vi "G# - StaticClassAndClassAttributes.vi"() -> ()   [LabVIEW 2020]
doc: "Static Classes and Class Attributes\nThis example demonstrates how static classes and class attributes works.\n\nBy using the G# Debugger found in Tools->G# Debugger a text log can be followed showing how the objects were created and destroyed."
uses:
  MyOrdinaryClass_class/MyOrdinaryClass.lvclass
  MyStaticClass_class/MyStaticClass.lvclass
  vi.lib/addons/_AddQ/G#Object/G#Object.lvclass
panel:
  in  "error in (no error)":errorcluster
  out "MyClassAttribute after garbage collector":dbl
  out "MyClassAttribute ordinary after garbage collector":string
  out "MyClassAttribute ordinary class unaffected by objects life cycle":string
  out "error out":errorcluster
  out "MyClassAttribute Ordinary Class":string
  out "MyClassAttribute Static Class":dbl
  # "Static Classes and Class Attributes\nThis example demonstrates how static classes and class attributes works.\n\nBy using the G# Debugger found in Tools->G# Debugger a text log can be followed showing how the objects were created and destroyed."
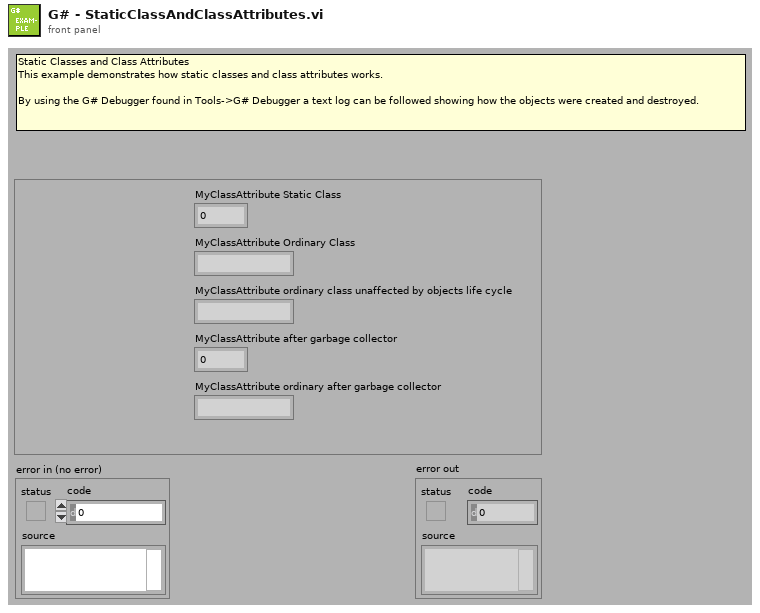
[diagram p1: front panel]
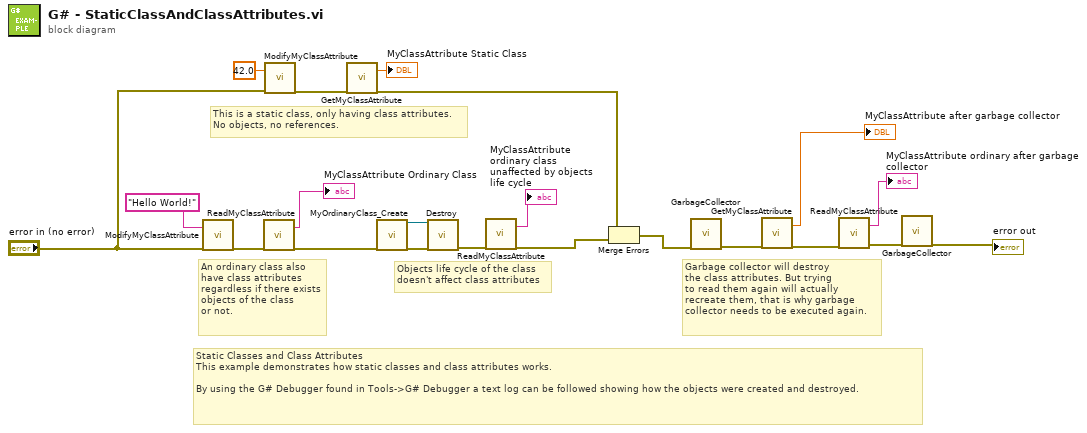
[diagram p0: block diagram]
diagram:
  # "Static Classes and Class Attributes\nThis example demonstrates how static classes and class attributes works.\n\nBy using the G# Debugger found in Tools->G# Debugger a text log can be followed showing how the objects were created and destroyed."
  # "Garbage collector will destroy\nthe class attributes. But trying\nto read them again will actually\nrecreate them, that is why garbage\ncollector needs to be executed again."
  # "Objects life cycle of the class\ndoesn't affect class attributes"
  # "An ordinary class also\nhave class attributes\nregardless if there exists\nobjects of the class\nor not."
  # "This is a static class, only having class attributes.\nNo objects, no references."
  n1 = call "ModifyMyClassAttribute.vi"("string"="Hello World!", "error in (no error)"="error in (no error)") -> ("error out"=w16:errorcluster)  [unwired: 17 in]
  n2 = call "ReadMyClassAttribute.vi"("error in (no error)"=w16) -> ("MyClassAttribute"=→"MyClassAttribute Ordinary Class":string, "error out"=w15:errorcluster)  [unwired: 17 in]
  n3 = call "ModifyMyClassAttribute.vi"("increment"=42.0, "error in (no error)"="error in (no error)") -> ("error out"=w19:errorcluster)  [unwired: 17 in]
  n4 = call "GetMyClassAttribute.vi"("error in (no error)"=w19) -> ("MyClassAttribute"=→"MyClassAttribute Static Class":dbl, "error out"=w17:errorcluster)  [unwired: 17 in]
  n5 = call "MyOrdinaryClass_Create.vi"("error in (no error)"=w15) -> ("reference out"=w13:refnum<class "MyOrdinaryClass.lvclass">, "error out"=w14:errorcluster)  [unwired: 17 in]
  n6 = call-dynamic "Destroy.vi"("reference in"=w13, "error in (no error)"=w14) -> ("error out"=w9:errorcluster)  [unwired: 16 in, 1 out]
  n7 = call "ReadMyClassAttribute.vi"("error in (no error)"=w9) -> ("MyClassAttribute"=→"MyClassAttribute ordinary class unaffected by objects life cycle":string, "error out"=w8:errorcluster)  [unwired: 17 in]
  n8 = Merge Errors(w17, w8) -> (w10:errorcluster)
  n9 = call "GarbageCollector.vi"("error in (no error)"=w10) -> ("error out"=w3:errorcluster)  [unwired: 16 in, 2 out]
  n10 = call "GetMyClassAttribute.vi"("error in (no error)"=w3) -> ("MyClassAttribute"=→"MyClassAttribute after garbage collector":dbl, "error out"=w2:errorcluster)  [unwired: 17 in]
  n11 = call "ReadMyClassAttribute.vi"("error in (no error)"=w2) -> ("MyClassAttribute"=→"MyClassAttribute ordinary after garbage collector":string, "error out"=w6:errorcluster)  [unwired: 17 in]
  n12 = call "GarbageCollector.vi"("error in (no error)"=w6) -> ("error out"=→"error out":errorcluster)  [unwired: 16 in, 2 out]
